vi "CalciumRecordings_github.vi"() -> ()   [LabVIEW 2014]
uses:
  <vilib>/Utility/error.llb/DialogType.ctl
  <vilib>/DAQmx/write.llb/DAQmx Write (Analog DBL 1Chan 1Samp).vi
  <vilib>/DAQmx/create/channels.llb/DAQmx Create Channel (AO-Voltage-Basic).vi
  <vilib>/measure/matone.llb/Extract Single Tone Information N Chan.vi
  <vilib>/DAQmx/miscellaneous.llb/DAQmx Fill In Error Info.vi
  <vilib>/measure/NI_MAPro.lvlib
panel:
  out "detected frequency":dbl[](array[numeric]) format="%.2p"
  in  "GAIN":dbl=0.2 format="%0.2f"
  in  "?":enum32{"stim", "Demodulated", "trigger"}(tab)
  out "ref":dynamicdata(graph)
  out "ref":dbl[](graph)
  out "?":dynamicdata(graph)
  in  "?":enum32{"Modulated", "Demodulated"}(tab)
  out "sig":dynamicdata(graph)
  out "sig":dbl[](graph)
  out "Ms timer value":u32
  in  "Enable":bool=TRUE
  out "Saving Data":bool
  in  "File Path":path
  out "DAQ number of loops":i32
  in  "?":bool
  # "Save Data"
  # "DEFAULT PATH:\nD:\\data\\2015\\test.lvm"
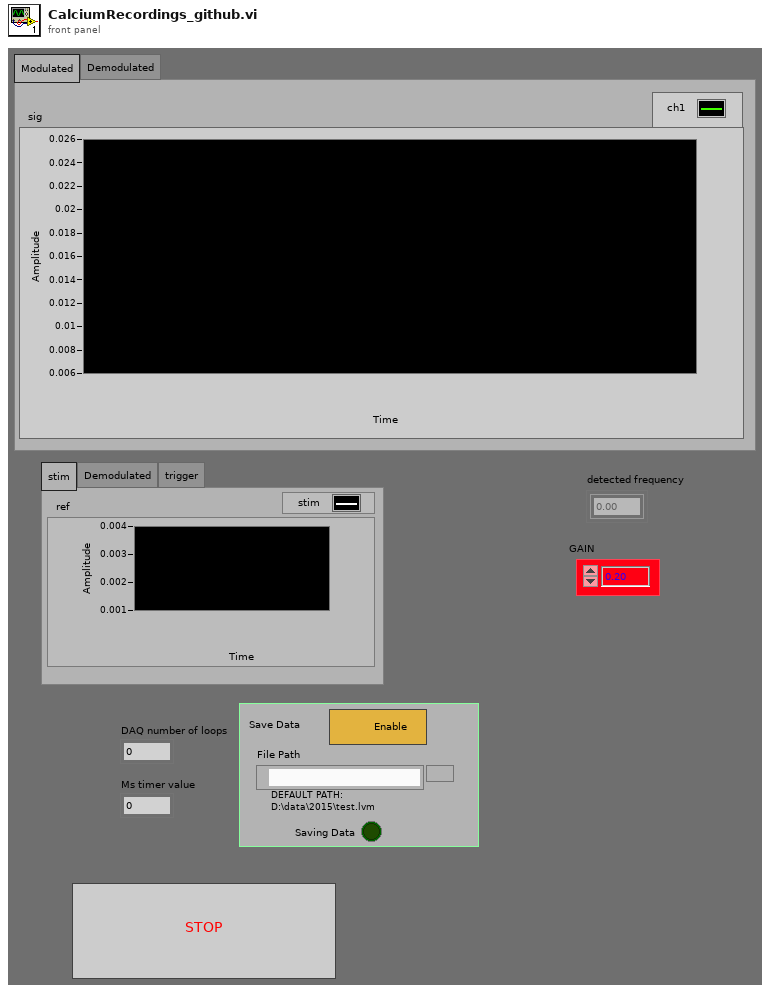
[diagram p1: front panel]
types:
  T1 = enum32{"none", "input signal", "detected signal", "residual signal"}
  T2 = typedef "DialogType.ctl" = u16
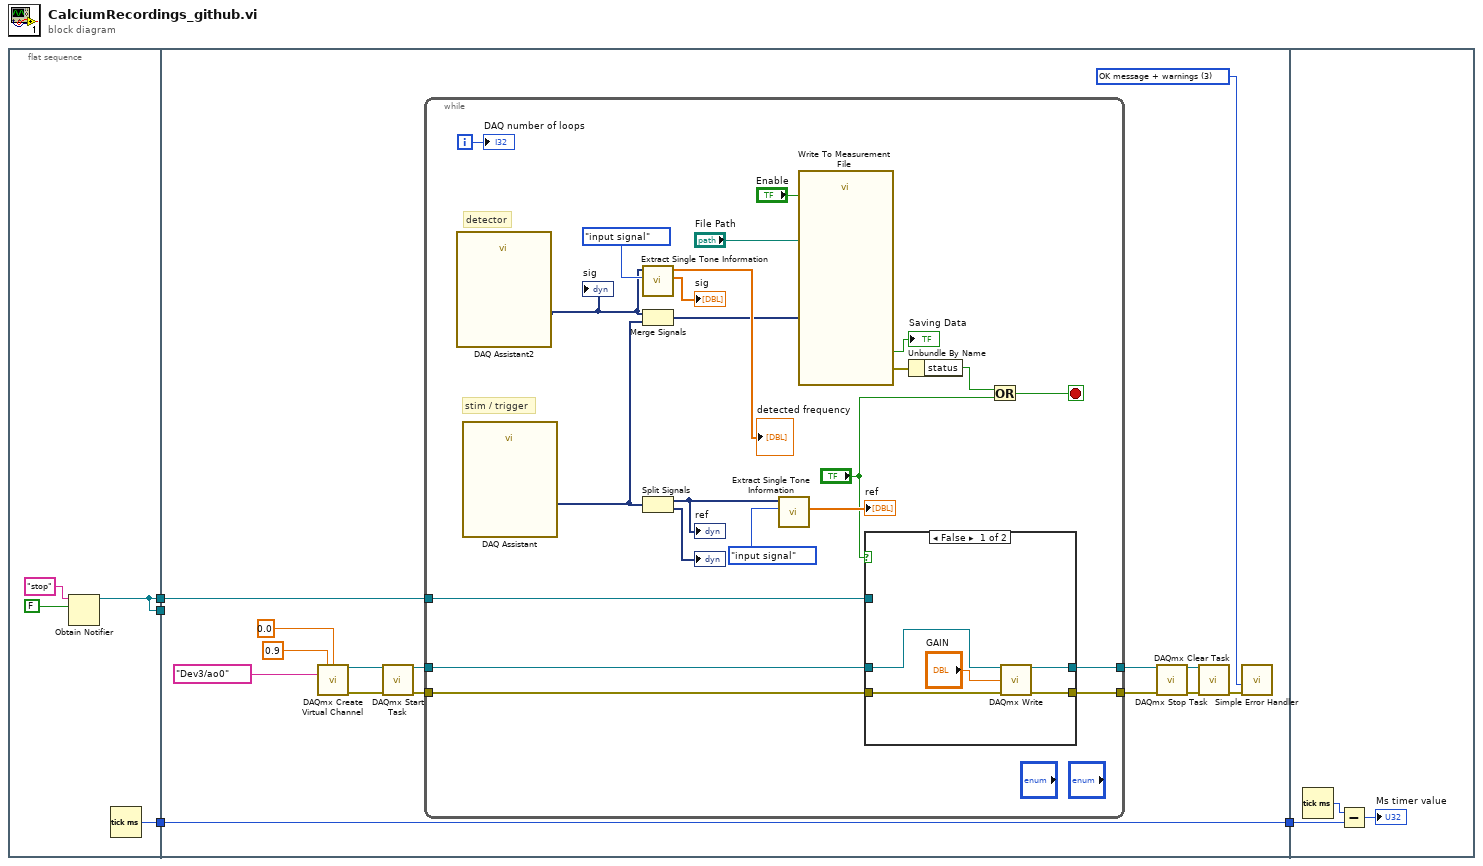
[diagram p0: block diagram]
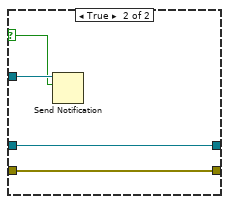
[diagram p2: hidden frame]
diagram:
  n1 = flat-sequence {
    tunnel: [w8] -> w4
    tunnel: [w6] -> w2
    tunnel: [w6] -> w1
    tunnel: w4 -> [w23]
    tunnel: [w23] -> w3
    tunnel: w2 -> [w22]
    tunnel: w1 -> [_]
    tunnel: w3 -> [w56]
    frame #0 {
      n2 = Obtain Notifier(name (unnamed)="stop", notification data type=FALSE ("if stop")) -> (notifier out=w6:refnum<notifier>)  [unwired: 2 in, 2 out]
      n3 = Tick Count (ms)() -> (millisecond timer value=w8:u32)
    }
    frame #1 {
      w14 = T2 3 items=["no dialog", "OK message", "continue or stop message", "OK message + warnings", "continue/stop + warnings"] ("type of dialog (OK msg:1)")
      n4 = call-poly <vilib>:"DAQmx Create Virtual Channel.vi"("maximum value"=0.9, "minimum value"=0.0, "physical channels"=tag "Dev3/ao0") -> ("task out"=w20:refnum<k21>, "error out"=w21:errorcluster)  [unwired: 11 in]
      n5 = call <vilib>:"DAQmx Start Task.vi"("task/channels in"=w20, "error in"=w21) -> ("task out"=w16:refnum<k21>, "error out"=w15:errorcluster)  [unwired: 12 in]
      n6 = while {
        tunnel: w22 -> [w39]
        tunnel: w16 -> [w33]
        tunnel: w15 -> [w32]
        tunnel: [w30] -> w10
        tunnel: [w31] -> w9
        i -> [w46]
        stop <- w41 stop-if-true
        # "stim / trigger"
        # "detector"
        n7 = call "DAQ Assistant2"() -> ("data"=w26:dynamicdata)  [unwired: 16 in, 3 out]
        "sig" <- w26
        n8 = call "DAQ Assistant"() -> ("data"=w25:dynamicdata)  [unwired: 16 in, 3 out]
        n9 = call-poly <vilib>:"Extract Single Tone Information.vi"("export mode"=T1."input signal", "time signals in"=w26) -> ("detected amplitudes"=→"sig":dbl[], "detected frequencies"=→"detected frequency":dbl[])  [unwired: 4 in, 4 out]
        n10 = Merge Signals(w26, w25) -> (w27:dynamicdata)
        n11 = Split Signals(w25) -> (w24:dynamicdata, →"?":dynamicdata)  [unwired: 2 in]
        "ref" <- w24
        n12 = call-poly <vilib>:"Extract Single Tone Information.vi"("export mode"=T1."input signal", "time signals in"=w24) -> ("detected amplitudes"=→"ref":dbl[])  [unwired: 4 in, 5 out]
        n13 = call "Write To Measurement File"("Signals"=w27, "Enable"="Enable", "Filename"="File Path") -> ("Saving Data"=→"Saving Data":bool, "error out"=w42:errorcluster)  [unwired: 14 in, 1 out]
        n14 = case shown="False" "?" {
          selector: "?" -> [_ w54]
          tunnel: w39 -> [_ w55]
          tunnel: w33 -> [w51 w52]
          tunnel: w32 -> [w50 w53]
          tunnel: [w49 w52] -> w31
          tunnel: [w48 w53] -> w30
          frame False {
            n15 = call-poly <vilib>:"DAQmx Write.vi"("task/channels in"=w51, "data"="GAIN", "error in"=w50) -> ("task out"=w49:refnum<k21>, "error out"=w48:errorcluster)  [unwired: 10 in, 1 out]
          }
          frame True {
            n16 = Send Notification(notification=w54, notifier=w55) -> ()  [unwired: 1 in, 2 out]
          }
        }
        n17 = Unbundle By Name(w42) -> ("status"=w40:bool)
        n18 = Or(x=w40, y="?") -> (x .or. y?=w41:bool)
        "DAQ number of loops" <- w46
      }
      n19 = call <vilib>:"DAQmx Stop Task.vi"("task/channels in"=w9, "error in"=w10) -> ("task out"=w12:refnum<k21>, "error out"=w13:errorcluster)  [unwired: 12 in]
      n20 = call <vilib>:"DAQmx Clear Task.vi"("task in"=w12, "error in"=w13) -> ("error out"=w11:errorcluster)  [unwired: 13 in]
      n21 = call <vilib>:"Simple Error Handler.vi"("type of dialog (OK msg:1)"=w14, "error in (no error)"=w11) -> ()  [unwired: 3 in, 5 out]
    }
    frame #2 {
      n22 = Tick Count (ms)() -> (millisecond timer value=w57:u32)
      n23 = Subtract(x=w57, y=w56) -> (x-y=→"Ms timer value":u32)
    }
  }
